vi "Refresh line clock.vi"(9 "line clock output":i32, 10 "Resolution":i32, 11 "Num of undershoot":i32) -> (3 "Refresh?":bool)   [LabVIEW 2015]
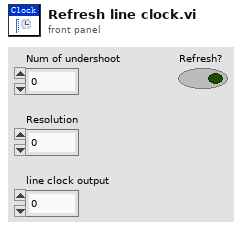
[diagram p1: front panel]
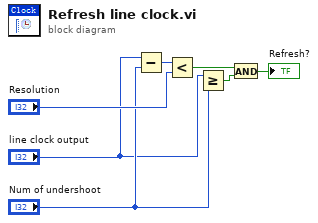
[diagram p0: block diagram]
diagram:
  n1 = Subtract(x="line clock output", y="Num of undershoot") -> (x-y=w2:i32)
  n2 = Less?(x=w2, y="Resolution") -> (x < y?=w3:bool)
  n3 = Greater Or Equal?(x="line clock output", y="Num of undershoot") -> (x >= y?=w4:bool)
  n4 = And(x=w3, y=w4) -> (x .and. y?=→"Refresh?":bool)
